vi "诊断标定4.vi"(8 "CAN端口":u16(ring), 9 "设备索引号":u16(ring), 10 "CAN卡类型":u32(ring)=4) -> ()   [LabVIEW 2013] (continued)
                  tunnel: w1914 -> [w1917 w1925]
                  tunnel: w1913 -> [w1916 w1924]
                  tunnel: w1912 -> [w1915 w1923]
                  tunnel: u8 137 ("命令") -> [_ w1922]
                  frame #0 {
                    n1213 = dll-call lib="PTH1Aabs EEV05EV05监控上位机-EV05EV05data\nusbcan.dll" fn="VCI_ClearBuffer"("DeviceType"=w1917, "DeviceInd"=w1916, "CANInd"=w1915) -> (error out=w1918:errorcluster)  [unwired: 4 in, 4 out]
                    n1214 = call <vilib>:"Clear Errors.vi"("error in (no error)"=w1918) -> ()  [unwired: 6 in, 1 out]
                  }
                  frame #1 {
                    w1921 = u32 2 ("命令序号")
                    n1215 = local read "从板板号"() -> (w1919:u8)
                    n1216 = local write "命令"(w1922) -> ()
                    n1217 = call "多帧发送机制(EV05).vi"("can卡类型"=w1925, "设备索引号"=w1924, "CAN端口"=w1923, "命令"=w1922, "板号"=w1919, "命令序号"=w1921, "输入数据"=dbl[] [0.0]) -> ()  [unwired: 1 in, 12 out]
                    n1218 = local write "命令序号"(w1921) -> ()
                  }
                }
              }
              frame #1 {
                n1219 = while {
                  tunnel: [w1927] -> w1926
                  i -> [w1932]
                  stop <- w1929 stop-if-true
                  n1220 = global read "EV05全局变量1.vi" "写入超时"() -> (w1927:bool)
                  n1221 = Greater Or Equal?(x=w1932, y=25) -> (x >= y?=w1930:bool)
                  n1222 = Or(x=w1927, y=w1930) -> (x .or. y?=w1929:bool)
                  n1223 = Wait Until Next ms Multiple(millisecond multiple=u32 100 ("毫秒倍数")) -> ()  [unwired: 1 out]
                }
              }
              frame #2 {
                n1224 = case shown="假" w1933 {
                  frame False {
                    n1225 = control-ref of="结果"() -> (w1936:refnum<vi>)
                    n1226 = Concatenate Strings("平台软件版本" ("字符串"), "     读取失败" ("字符串")) -> (w1938:string)
                    n1227 = Build Array(w1938) -> (w1935:string[])
                    n1228 = call "表格编辑(版本读取).vi"("新元素/子数组"=w1935, "活动单元格:单元格背景色"=u32 16740749, "MCListbox引用句柄"=w1936) -> ()  [unwired: 9 out]
                  }
                  frame True {
                  }
                }
                n1229 = call <vilib>:"Unset Busy.vi"() -> ()  [unwired: 2 in, 10 out]
              }
            }
          }
          frame "模块软件版本读取" {
            n1230 = local read "模块软件版本"() -> (w1941:T16)
            n1231 = local read "从板板号"() -> (w1940:u8)
            n1232 = case shown="\"全部读取\"" w1941 {
              selector: w1941 -> [w1942 w1986]
              tunnel: w1940 -> [_ w1985]
              frame "BCUMCAL", Default {
                n1233 = stacked-sequence {
                  seq-local: [_ _ w1968 _] -> [_ _ _ w1975]
                  tunnel: w1942 -> [_ w1948 _ w1976]
                  frame #0 {
                    w1947 = FALSE ("写?")
                    n1234 = call <vilib>:"Set Busy.vi"("disable click? (T)"=FALSE) -> ()  [unwired: 3 in, 8 out]
                    n1235 = local write "写?"(w1947) -> ()
                    n1236 = global write "EV05全局变量1.vi" "流控帧 2"(TRUE ("流控帧 2")) -> ()
                    n1237 = global write "EV05全局变量1.vi" "写入超时"(w1947) -> ()
                    n1238 = local write "控制1"(TRUE ("控制1")) -> ()
                    n1239 = local write "消除"(TRUE ("消除")) -> ()
                  }
                  frame #1 {
                    n1240 = Quotient & Remainder(x=w1948, y=256) -> (x-y*floor(x/y)=w1949:i32, floor(x/y)=w1950:i32)
                    n1241 = Build Array(w1950, w1949, u8 0 ("板号")) -> (w1953:i32[])
                    n1242 = local read "设备索引号"() -> (w1955:u16)
                    n1243 = local read "CAN卡类型"() -> (w1956:u32)
                    n1244 = local read "CAN端口"() -> (w1954:u16)
                    n1245 = stacked-sequence {
                      tunnel: w1956 -> [w1959 w1967]
                      tunnel: w1955 -> [w1958 w1966]
                      tunnel: w1954 -> [w1957 w1965]
                      tunnel: w1953 -> [_ w1964]
                      frame #0 {
                        n1246 = dll-call lib="PTH1Aabs EEV05EV05监控上位机-EV05EV05data\nusbcan.dll" fn="VCI_ClearBuffer"("DeviceType"=w1959, "DeviceInd"=w1958, "CANInd"=w1957) -> (error out=w1960:errorcluster)  [unwired: 4 in, 4 out]
                        n1247 = call <vilib>:"Clear Errors.vi"("error in (no error)"=w1960) -> ()  [unwired: 6 in, 1 out]
                      }
                      frame #1 {
                        w1963 = u8 137 ("命令")
                        w1961 = u32 3 ("命令序号")
                        n1248 = local read "从板板号"() -> (w1962:u8)
                        n1249 = local write "命令"(w1963) -> ()
                        n1250 = call "多帧发送机制(EV05).vi"("can卡类型"=w1967, "设备索引号"=w1966, "CAN端口"=w1965, "命令"=w1963, "板号"=w1962, "命令序号"=w1961, "输入数据"=w1964) -> ()  [unwired: 1 in, 12 out]
                        n1251 = local write "命令序号"(w1961) -> ()
                      }
                    }
                  }
                  frame #2 {
                    n1252 = while {
                      tunnel: [w1969] -> w1968
                      i -> [w1974]
                      stop <- w1970 stop-if-true
                      n1253 = global read "EV05全局变量1.vi" "写入超时"() -> (w1969:bool)
                      n1254 = Greater Or Equal?(x=w1974, y=25) -> (x >= y?=w1971:bool)
                      n1255 = Or(x=w1969, y=w1971) -> (x .or. y?=w1970:bool)
                      n1256 = Wait Until Next ms Multiple(millisecond multiple=u32 100 ("毫秒倍数")) -> ()  [unwired: 1 out]
                    }
                  }
                  frame #3 {
                    n1257 = call <vilib>:"Unset Busy.vi"() -> ()  [unwired: 2 in, 10 out]
                    n1258 = case shown="假" w1975 {
                      tunnel: w1976 -> [w1978 _]
                      frame False {
                        n1259 = Number To Decimal String(number=w1978) -> (decimal integer string=w1979:string)  [unwired: 1 out]
                        n1260 = control-ref of="结果"() -> (w1980:refnum<vi>)
                        n1261 = Concatenate Strings("模块" ("字符串"), w1979, "     读取失败" ("字符串")) -> (w1983:string)
                        n1262 = Build Array(w1983) -> (w1982:string[])
                        n1263 = call "表格编辑(版本读取).vi"("新元素/子数组"=w1982, "活动单元格:单元格背景色"=u32 16740749, "MCListbox引用句柄"=w1980) -> ()  [unwired: 9 out]
                      }
                      frame True {
                      }
                    }
                  }
                }
              }
              frame "全部读取" {
                n1264 = stacked-sequence {
                  seq-local: [w1987 _] -> [_ w2025]
                  tunnel: w1986 -> [_ w2027]
                  tunnel: w1985 -> [w1988 w2026]
                  frame #0 {
                    n1265 = stacked-sequence {
                      tunnel: w1988 -> [_ w1997 _]
                      tunnel: [_ _ w2017] -> w1987
                      frame #0 {
                        w1993 = FALSE ("写?")
                        n1266 = control-ref of="模块软件版本"() -> (w1991:refnum<vi>)
                        n1267 = call <vilib>:"Set Busy.vi"("disable click? (T)"=FALSE) -> ()  [unwired: 3 in, 8 out]
                        n1268 = local write "写?"(w1993) -> ()
                        n1269 = property class="MCListbox (严格)"(reference=w1991, "ItemNames"=string[][] []) -> ()  [unwired: 1 in, 2 out]
                        n1270 = global write "EV05全局变量1.vi" "写入超时"(w1993) -> ()
                        n1271 = global write "EV05全局变量1.vi" "流控帧 2"(TRUE ("流控帧 2")) -> ()
                        n1272 = local write "消除"(TRUE ("消除")) -> ()
                        n1273 = local write "控制1"(TRUE ("控制1")) -> ()
                        n1274 = local write "MODEL号"(u8[] [] ("MODEL号")) -> ()
                      }
                      frame #1 {
                        n1275 = local read "设备索引号"() -> (w1999:u16)
                        n1276 = local read "CAN卡类型"() -> (w2000:u32)
                        n1277 = local read "CAN端口"() -> (w1998:u16)
                        n1278 = stacked-sequence {
                          tunnel: w2000 -> [w2003 w2016]
                          tunnel: w1999 -> [w2002 w2015]
                          tunnel: w1998 -> [w2001 w2014]
                          tunnel: w1997 -> [_ w2006]
                          frame #0 {
                            n1279 = dll-call lib="PTH1Aabs EEV05EV05监控上位机-EV05EV05data\nusbcan.dll" fn="VCI_ClearBuffer"("DeviceType"=w2003, "DeviceInd"=w2002, "CANInd"=w2001) -> (error out=w2004:errorcluster)  [unwired: 4 in, 4 out]
                            n1280 = call <vilib>:"Clear Errors.vi"("error in (no error)"=w2004) -> ()  [unwired: 6 in, 1 out]
                          }
                          frame #1 {
                            w2012 = u8 137 ("命令")
                            w2010 = u32 3 ("命令序号")
                            n1281 = Quotient & Remainder(x=u8 0 ("板号"), y=256) -> (x-y*floor(x/y)=w2007:i32, floor(x/y)=w2008:i32)
                            n1282 = local write "命令"(w2012) -> ()
                            n1283 = Build Array(w2008, w2007, u8 0 ("板号")) -> (w2013:i32[])
                            n1284 = call "多帧发送机制(EV05).vi"("can卡类型"=w2016, "设备索引号"=w2015, "CAN端口"=w2014, "命令"=w2012, "板号"=w2006, "命令序号"=w2010, "输入数据"=w2013) -> ()  [unwired: 1 in, 12 out]
                            n1285 = local write "命令序号"(w2010) -> ()
                          }
                        }
                      }
                      frame #2 {
                        n1286 = while {
                          tunnel: [w2019] -> w2017
                          i -> [w2023]
                          stop <- w2020 stop-if-true
                          n1287 = local read "整车CAN测试"() -> (w2018:bool)
                          n1288 = global read "EV05全局变量1.vi" "写入超时"() -> (w2019:bool)
                          n1289 = Greater Or Equal?(x=w2023, y=35) -> (x >= y?=w2021:bool)
                          n1290 = Compound Arithmetic op=OR(w2018, w2019, w2021) -> (w2020:bool)
                          n1291 = Wait Until Next ms Multiple(millisecond multiple=u32 100 ("毫秒倍数")) -> ()  [unwired: 1 out]
                        }
                      }
                    }
                  }
                  frame #1 {
                    n1292 = case shown="真" w2025 {
                      tunnel: w2027 -> [_ w2037]
                      tunnel: w2026 -> [_ w2036]
                      frame False {
                        n1293 = control-ref of="结果"() -> (w2029:refnum<vi>)
                        n1294 = Concatenate Strings("模块编号" ("字符串"), "读取失败" ("字符串")) -> (w2032:string)
                        n1295 = Build Array(w2032) -> (w2031:string[])
                        n1296 = call "表格编辑(版本读取).vi"("新元素/子数组"=w2031, "活动单元格:单元格背景色"=u32 16740749, "MCListbox引用句柄"=w2029) -> ()  [unwired: 9 out]
                        n1297 = call <vilib>:"Unset Busy.vi"() -> ()  [unwired: 11 in, 1 out]
                      }
                      frame True {
                        n1298 = local read "MODEL号"() -> (w2035:u8[])
                        n1299 = Array Size(array=w2035) -> (size(s)=w2034:i32)
                        n1300 = for {
                          tunnel: w2037 -> [_]
                          tunnel: w2036 -> [w2040]
                          tunnel: w2035 -> [w2039] mode=indexing
                          tunnel: w2034 -> [w2038]
                          i -> [w2042]
                          n1301 = Increment(x=w2042) -> (x+1=w2041:i32)
                          n1302 = stacked-sequence {
                            seq-local: [_ _ _ w2069 _ _] -> [_ _ _ _ w2078 _]
                            seq-local: [_ w2048 _ _ _ _] -> [_ _ _ _ w2077 _]
                            tunnel: w2041 -> [_ _ _ _ _ w2089]
                            tunnel: w2039 -> [_ w2048 _ _ _ _]
                            tunnel: w2040 -> [_ w2049 _ _ _ _]
                            tunnel: w2038 -> [_ _ _ _ _ w2087]
                            frame #0 {
                              w2044 = FALSE ("写?")
                              n1303 = call <vilib>:"Set Busy.vi"("disable click? (T)"=FALSE) -> ()  [unwired: 3 in, 8 out]
                              n1304 = local write "写?"(w2044) -> ()
                              n1305 = global write "EV05全局变量1.vi" "写入超时"(w2044) -> ()
                              n1306 = global write "EV05全局变量1.vi" "流控帧 2"(TRUE ("流控帧 2")) -> ()
                              n1307 = local write "控制1"(TRUE ("控制1")) -> ()
                              n1308 = local write "消除"(TRUE ("消除")) -> ()
                            }
                            frame #1 {
                              n1309 = local read "设备索引号"() -> (w2051:u16)
                              n1310 = local read "CAN卡类型"() -> (w2052:u32)
                              n1311 = local read "CAN端口"() -> (w2050:u16)
                              n1312 = stacked-sequence {
                                tunnel: w2052 -> [w2055 w2068]
                                tunnel: w2051 -> [w2054 w2067]
                                tunnel: w2050 -> [w2053 w2066]
                                tunnel: w2049 -> [_ w2058]
                                tunnel: w2048 -> [_ w2057]
                                frame #0 {
                                n1313 = dll-call lib="PTH1Aabs EEV05EV05监控上位机-EV05EV05data\nusbcan.dll" fn="VCI_ClearBuffer"("DeviceType"=w2055, "DeviceInd"=w2054, "CANInd"=w2053) -> (error out=w2056:errorcluster)  [unwired: 4 in, 4 out]
                                n1314 = call <vilib>:"Clear Errors.vi"("error in (no error)"=w2056) -> ()  [unwired: 6 in, 1 out]
                                }
                                frame #1 {
                                w2064 = u8 137 ("命令")
                                w2062 = u32 3 ("命令序号")
                                n1315 = Quotient & Remainder(x=w2057, y=256) -> (x-y*floor(x/y)=w2059:i32, floor(x/y)=w2060:i32)
                                n1316 = local write "命令"(w2064) -> ()
                                n1317 = Build Array(w2060, w2059, u8 0 ("板号")) -> (w2065:i32[])
                                n1318 = call "多帧发送机制(EV05).vi"("can卡类型"=w2068, "设备索引号"=w2067, "CAN端口"=w2066, "命令"=w2064, "板号"=w2058, "命令序号"=w2062, "输入数据"=w2065) -> ()  [unwired: 1 in, 12 out]
                                n1319 = local write "命令序号"(w2062) -> ()
                                }
                              }
                            }
                            frame #2 {
                            }
                            frame #3 {
                              n1320 = while {
                                tunnel: [w2071] -> w2069
                                i -> [w2075]
                                stop <- w2072 stop-if-true
                                n1321 = local read "整车CAN测试"() -> (w2070:bool)
                                n1322 = global read "EV05全局变量1.vi" "写入超时"() -> (w2071:bool)
                                n1323 = Greater Or Equal?(x=w2075, y=25) -> (x >= y?=w2073:bool)
                                n1324 = Compound Arithmetic op=OR(w2070, w2071, w2073) -> (w2072:bool)
                                n1325 = Wait Until Next ms Multiple(millisecond multiple=u32 100 ("毫秒倍数")) -> ()  [unwired: 1 out]
                              }
                            }
                            frame #4 {
                              n1326 = call <vilib>:"Unset Busy.vi"() -> ()  [unwired: 11 in, 1 out]
                              n1327 = case shown="假" w2078 {
                                tunnel: w2077 -> [w2080 _]
                                frame False {
                                n1328 = control-ref of="结果"() -> (w2082:refnum<vi>)
                                n1329 = Number To Decimal String(number=w2080) -> (decimal integer string=w2081:string)  [unwired: 1 out]
                                n1330 = Concatenate Strings("模块" ("字符串"), w2081, "     读取失败" ("字符串")) -> (w2085:string)
                                n1331 = Build Array(w2085) -> (w2084:string[])
                                n1332 = call "表格编辑(版本读取).vi"("新元素/子数组"=w2084, "活动单元格:单元格背景色"=u32 16740749, "MCListbox引用句柄"=w2082) -> ()  [unwired: 9 out]
                                }
                                frame True {
                                }
                              }
                            }
                            frame #5 {
                              n1333 = Equal?(x=w2087, y=w2089) -> (x = y?=w2088:bool)
                              n1334 = case shown="真" w2088 {
                                frame False {
                                }
                                frame True {
                                n1335 = control-ref of="模块软件版本"() -> (w2100:refnum<vi>)
                                n1336 = local read "模块版本名称"() -> (w2099:string[][])
                                n1337 = local read "模块版本值"() -> (w2095:string[][])
                                n1338 = control-ref of="结果"() -> (w2107:refnum<vi>)
                                n1339 = property class="MCListbox (严格)"(reference=w2100) -> ("ItemNames"=w2103:string[][])  [unwired: 1 in, 2 out]
                                n1340 = local read "从板板号"() -> (w2090:u8)
                                n1341 = Concatenate Strings("模块版本读取完成" ("字符串")) -> (w2110:string)
                                n1342 = Build Array(w2110) -> (w2109:string[])
                                n1343 = call "表格编辑(版本读取).vi"("新元素/子数组"=w2109, "活动单元格:单元格背景色"=u32 21937, "MCListbox引用句柄"=w2107) -> ()  [unwired: 9 out]
                                n1344 = Transpose 2D Array(2D array=w2103) -> (transposed array=w2104:string[][])
                                n1345 = local read "模块个数"() -> (w2093:u8[])
                                n1346 = local write "整车CAN测试"(FALSE ("强制停止 2")) -> ()
                                n1347 = Index Array(array=w2104, index (row) #1=0 ("索引 (行)"), index (row) #2=1 ("索引 (行)")) -> (element #1=w2094:string[], element #2=w2096:string[])  [unwired: 2 in]
                                n1348 = Replace Array Subset(array=w2099, new element=w2094, index (row)=w2090) -> (w2098:string[][])  [unwired: 1 in]
                                n1349 = Replace Array Subset(array=w2095, new element=w2096, index (row)=w2090) -> (w2097:string[][])  [unwired: 1 in]
                                n1350 = local write "模块版本名称"(w2098) -> ()
                                n1351 = local write "模块版本值"(w2097) -> ()
                                n1352 = Array Size(array=w2094) -> (size(s)=w2091:i32)
                                n1353 = Replace Array Subset(array=w2093, new element=w2091, index=w2090) -> (w2092:u8[])
                                n1354 = local write "模块个数"(w2092) -> ()
                                }
                              }
                            }
                          }
                        }
                      }
                    }
                  }
                }
              }
            }
          }
          frame "硬件版本读取" {
            n1355 = stacked-sequence {
              seq-local: [_ _ w2118 _] -> [_ _ _ w2125]
              frame #0 {
                w2114 = u8 137 ("命令")
                w2113 = u32 4 ("命令序号")
                n1356 = local read "设备索引号"() -> (w2116:u16)
                n1357 = local read "CAN卡类型"() -> (w2117:u32)
                n1358 = local read "CAN端口"() -> (w2115:u16)
                n1359 = local read "从板板号"() -> (w2111:u8)
                n1360 = local write "命令"(w2114) -> ()
                n1361 = call "多帧发送机制(EV05).vi"("can卡类型"=w2117, "设备索引号"=w2116, "CAN端口"=w2115, "命令"=w2114, "板号"=w2111, "命令序号"=w2113, "输入数据"=dbl[] [0.0]) -> ()  [unwired: 1 in, 12 out]
                n1362 = local write "命令序号"(w2113) -> ()
              }
              frame #1 {
              }
              frame #2 {
                n1363 = while {
                  tunnel: [w2119] -> w2118
                  i -> [w2124]
                  stop <- w2120 stop-if-true
                  n1364 = global read "EV05全局变量1.vi" "写入超时"() -> (w2119:bool)
                  n1365 = Greater Or Equal?(x=w2124, y=25) -> (x >= y?=w2121:bool)
                  n1366 = Or(x=w2119, y=w2121) -> (x .or. y?=w2120:bool)
                  n1367 = Wait Until Next ms Multiple(millisecond multiple=u32 100 ("毫秒倍数")) -> ()  [unwired: 1 out]
                }
              }
              frame #3 {
                n1368 = case shown="假" w2125 {
                  frame False {
                    n1369 = control-ref of="结果"() -> (w2127:refnum<vi>)
                    n1370 = Concatenate Strings("硬件版本" ("字符串"), "     读取失败" ("字符串")) -> (w2130:string)
                    n1371 = Build Array(w2130) -> (w2129:string[])
                    n1372 = call "表格编辑(版本读取).vi"("新元素/子数组"=w2129, "活动单元格:单元格背景色"=u32 16740749, "MCListbox引用句柄"=w2127) -> ()  [unwired: 9 out]
                  }
                  frame True {
                  }
                }
                n1373 = call <vilib>:"Unset Busy.vi"() -> ()  [unwired: 2 in, 10 out]
              }
            }
          }
          frame "写配置文件" {
            n1374 = disable-structure shown="启用" {
              frame Enabled {
                n1375 = local read "主从选择"() -> (w2138:enum32{"主板", "从板"})
                n1376 = case shown="\"从板\"" w2138 {
                  tunnel: [w2156 w2339] -> w2141
                  tunnel: ["M0" w2345] -> w2139
                  frame "主板", Default {
                    n1377 = stacked-sequence {
                      seq-local: [w2161 _ _ _ _ _ _] -> [_ w2190 _ _ _ _ _]
                      seq-local: [string[] ["电池额定容量", "电池实际容量", "SOC", "SOH", "车牌号", "配置文件版本", "产品编号", "系统时钟"] _ _ _ _ _ _] -> [_ w2192 _ _ _ _ _]
                      seq-local: [_ _ _ _ string[] ["风机开启温度", "风机关闭温度", "加热开启温度", "加热关闭温度", "风机开启温差", "风机关闭温差", "加热关闭温差"] _ _] -> [_ _ _ _ _ w2291 _]
                      seq-local: [_ _ _ _ w2272 _ _] -> [_ _ _ _ _ w2289 _]
                      tunnel: [w2162 _ _ _ _ _ _] -> w2158
                      tunnel: [_ w2193 _ _ _ _ _] -> w2155
                      tunnel: [_ _ w2217 _ _ _ _] -> w2154
                      tunnel: [_ _ _ w2244 _ _ _] -> w2153
                      tunnel: [_ _ _ _ _ w2292 _] -> w2152
                      tunnel: [_ _ _ _ _ _ w2309] -> w2151
                      frame #0 {
                        n1378 = local read "从板个数"() -> (w2181:dbl)
                        n1379 = control-ref of="项目信息"() -> (w2182:refnum<vi>)
                        n1380 = control-ref of="项目信息2"() -> (w2175:refnum<vi>)
                        n1381 = property class="Clust (严格)"(reference=w2175) -> ("Value"=w2174:T8)  [unwired: 1 in, 2 out]
                        n1382 = property class="Tbl (严格)"(reference=w2182) -> ("Value"=w2178:string[][])  [unwired: 1 in, 2 out]
                        n1383 = Number To Decimal String(number=w2181) -> (decimal integer string=w2180:string)  [unwired: 1 out]
                        n1384 = Unbundle(w2174) -> ("电池额定容量(A)"=w2173:dbl, "电池实际容量(A)"=w2172:dbl, "车架(牌)号"=w2170:string, "配置文件版本"=w2169:string, "SOH(%)"=w2164:dbl, "SOC(%)"=w2163:dbl, "产品编号"=w2168:string, "系统时钟"=w2167:string)  [unwired: 1 out]
                        n1385 = Build Array("从板个数" ("元素"), w2180) -> (w2176:string[])
                        n1386 = Build Array(w2173, w2172, w2163, w2164) -> (w2171:dbl[])
                        n1387 = Build Array(w2170, w2169, w2168, w2167) -> (w2165:string[])
                        n1388 = Insert Into Array(array=w2178, index (row)=0 ("索引 (行)"), new element=w2176) -> (w2162:string[][])  [unwired: 1 in]
                        n1389 = for {
                          tunnel: w2171 -> [w2184] mode=indexing
                          tunnel: [w2183] -> w2166 mode=indexing
                          n1390 = Format Into String(format string="%#f" ("格式字符串"), w2184) -> (resulting string=w2183:string)  [unwired: 2 in, 1 out]
                        }
                        n1391 = Insert Into Array(array=w2166, new element=w2165) -> (w2161:string[])  [unwired: 1 in]
                      }
                      frame #1 {
                        n1392 = control-ref of="一级故障"() -> (w2213:refnum<vi>)
                        n1393 = property class="Clust (严格)"(reference=w2213) -> ("Value"=w2212:T9)  [unwired: 1 in, 2 out]
                        n1394 = Unbundle(w2212) -> ("总电压过高"=w2211:dbl, "整组电压不均衡"=w2206:dbl, "SOC过高"=w2199:dbl, "单体电压过高"=w2202:dbl, "总电压过低"=w2210:dbl, "温度过高"=w2209:dbl, "温度过低"=w2208:dbl, "单组电压不均衡"=w2207:dbl, "整组温度不均衡"=w2204:dbl, "单组温度不均衡"=w2205:dbl, "单体电压过低"=w2203:dbl, "充电电流过高"=w2201:dbl, "放电电流过高"=w2200:dbl, "SOC过低"=w2198:dbl, "内阻过大"=w2197:dbl, "极柱温度过高"=w2196:dbl, "SOH过低"=w2195:dbl)
                        n1395 = Build Array(w2211, w2210, w2209, w2208, w2207, w2206, w2205, w2204, w2202, w2203, w2201, w2200, w2199, w2198, w2197, w2196, w2195) -> (w2194:dbl[])
                        n1396 = for {
                          tunnel: w2194 -> [w2215] mode=indexing
                          tunnel: [w2214] -> w2189 mode=indexing
                          n1397 = Format Into String(format string="%#f" ("格式字符串"), w2215) -> (resulting string=w2214:string)  [unwired: 2 in, 1 out]
                        }
                        n1398 = Insert Into Array(array=w2190, new element=w2189) -> (w2188:string[])  [unwired: 1 in]
                        n1399 = Insert Into Array(array=w2192, new element=string[] ["总电压过高一级", "总电压过低一级", "温度过高一级", "温度过低一级", "单组电压不均衡一级", "整组电压不均衡一级", "单组温度不均衡一级", "整组温度不均衡一级", "单体电压过高一级", "单体电压过低一级", "充电电流过高一级", "放电电流过高一级", "SOC过高一级", "SOC过低一级", "内阻过大一级", "极柱温度过高一级", "SOH过低一级"]) -> (w2187:string[])  [unwired: 1 in]
                        n1400 = Build Array(w2187, w2188) -> (w2186:string[][])
                        n1401 = Transpose 2D Array(2D array=w2186) -> (transposed array=w2193:string[][])
                      }
                      frame #2 {
                        n1402 = control-ref of="一级故障 2"() -> (w2218:refnum<vi>)
                        n1403 = property class="Clust (严格)"(reference=w2218) -> ("Value"=w2240:T9)  [unwired: 1 in, 2 out]
                        n1404 = Unbundle(w2240) -> ("总电压过高"=w2239:dbl, "整组电压不均衡"=w2234:dbl, "SOC过高"=w2227:dbl, "单体电压过高"=w2230:dbl, "总电压过低"=w2238:dbl, "温度过高"=w2237:dbl, "温度过低"=w2236:dbl, "单组电压不均衡"=w2235:dbl, "整组温度不均衡"=w2232:dbl, "单组温度不均衡"=w2233:dbl, "单体电压过低"=w2231:dbl, "充电电流过高"=w2229:dbl, "放电电流过高"=w2228:dbl, "SOC过低"=w2226:dbl, "内阻过大"=w2225:dbl, "极柱温度过高"=w2224:dbl, "SOH过低"=w2223:dbl)
                        n1405 = Build Array(w2239, w2238, w2237, w2236, w2235, w2234, w2233, w2232, w2230, w2231, w2229, w2228, w2227, w2226, w2225, w2224, w2223) -> (w2222:dbl[])
                        n1406 = for {
                          tunnel: w2222 -> [w2242] mode=indexing
                          tunnel: [w2241] -> w2221 mode=indexing
                          n1407 = Format Into String(format string="%#f" ("格式字符串"), w2242) -> (resulting string=w2241:string)  [unwired: 2 in, 1 out]
                        }
                        n1408 = Build Array(string[] ["总电压过高二级", "总电压过低二级", "温度过高二级", "温度过低二级", "单组电压不均衡二级", "整组电压不均衡二级", "单组温度不均衡二级", "整组温度不均衡二级", "单体电压过高二级", "单体电压过低二级", "充电电流过高二级", "放电电流过高二级", "SOC过高二级", "SOC过低二级", "内阻过大二级", "极柱温度过高二级", "SOH过低二级"], w2221) -> (w2219:string[][])
                        n1409 = Transpose 2D Array(2D array=w2219) -> (transposed array=w2217:string[][])
                      }
                      frame #3 {
                        n1410 = control-ref of="一级故障 3"() -> (w2245:refnum<vi>)
                        n1411 = property class="Clust (严格)"(reference=w2245) -> ("Value"=w2267:T9)  [unwired: 1 in, 2 out]
                        n1412 = Unbundle(w2267) -> ("总电压过高"=w2266:dbl, "整组电压不均衡"=w2261:dbl, "SOC过高"=w2254:dbl, "单体电压过高"=w2257:dbl, "总电压过低"=w2265:dbl, "温度过高"=w2264:dbl, "温度过低"=w2263:dbl, "单组电压不均衡"=w2262:dbl, "整组温度不均衡"=w2259:dbl, "单组温度不均衡"=w2260:dbl, "单体电压过低"=w2258:dbl, "充电电流过高"=w2256:dbl, "放电电流过高"=w2255:dbl, "SOC过低"=w2253:dbl, "内阻过大"=w2252:dbl, "极柱温度过高"=w2251:dbl, "SOH过低"=w2250:dbl)
                        n1413 = Build Array(w2266, w2265, w2264, w2263, w2262, w2261, w2260, w2259, w2257, w2258, w2256, w2255, w2254, w2253, w2252, w2251, w2250) -> (w2249:dbl[])
                        n1414 = for {
                          tunnel: w2249 -> [w2269] mode=indexing
                          tunnel: [w2268] -> w2248 mode=indexing
                          n1415 = Format Into String(format string="%#f" ("格式字符串"), w2269) -> (resulting string=w2268:string)  [unwired: 2 in, 1 out]
                        }
                        n1416 = Build Array(string[] ["总电压过高三级", "总电压过低三级", "温度过高三级", "温度过低三级", "单组电压不均衡三级", "整组电压不均衡三级", "单组温度不均衡三级", "整组温度不均衡三级", "单体电压过高三级", "单体电压过低三级", "充电电流过高三级", "放电电流过高三级", "SOC过高三级", "SOC过低三级", "内阻过大三级", "极柱温度过高三级", "SOH过低三级"], w2248) -> (w2246:string[][])
                        n1417 = Transpose 2D Array(2D array=w2246) -> (transposed array=w2244:string[][])
                      }
                      frame #4 {
                        n1418 = control-ref of="加热控制参数"() -> (w2282:refnum<vi>)
                        n1419 = property class="Clust (严格)"(reference=w2282) -> ("Value"=w2281:T10)  [unwired: 1 in, 2 out]
                        n1420 = Unbundle(w2281) -> ("风机开启温度"=w2280:dbl, "风机关闭温度"=w2279:dbl, "加热开启温度"=w2278:dbl, "加热关闭温度"=w2277:dbl, "风机开启温差"=w2276:dbl, "风机关闭温差"=w2275:dbl, "加热关闭温差"=w2271:dbl)
                        n1421 = Build Array(w2280, w2279, w2278, w2277, w2276, w2275, w2271) -> (w2274:dbl[])
                        n1422 = for {
                          tunnel: w2274 -> [w2284] mode=indexing
                          tunnel: [w2283] -> w2272 mode=indexing
                          n1423 = Format Into String(format string="%#f" ("格式字符串"), w2284) -> (resulting string=w2283:string)  [unwired: 2 in, 1 out]
                        }
                      }
                      frame #5 {
                        n1424 = control-ref of="充电控制参数"() -> (w2302:refnum<vi>)
                        n1425 = property class="Clust (严格)"(reference=w2302) -> ("Value"=w2304:T11)  [unwired: 1 in, 2 out]
                        n1426 = Unbundle(w2304) -> ("最大允许单体电压"=w2301:dbl, "最大允许总电压"=w2300:dbl, "最小允许单体电压"=w2299:dbl, "最大允许充电电流"=w2298:dbl, "最小允许充电电流"=w2297:dbl, "最大允许充电温度"=w2296:dbl, "最小允许充电温度"=w2295:dbl, "电流步长"=w2294:dbl)
                        n1427 = Build Array(w2301, w2300, w2299, w2298, w2297, w2296, w2295, w2294) -> (w2303:dbl[])
                        n1428 = for {
                          tunnel: w2303 -> [w2306] mode=indexing
                          tunnel: [w2305] -> w2288 mode=indexing
                          n1429 = Format Into String(format string="%#f" ("格式字符串"), w2306) -> (resulting string=w2305:string)  [unwired: 2 in, 1 out]
                        }
                        n1430 = Insert Into Array(array=w2289, new element=w2288) -> (w2287:string[])  [unwired: 1 in]
                        n1431 = Insert Into Array(array=w2291, new element=string[] ["最大允许单体电压", "最大允许总电压", "最小允许单体电压", "最大允许充电电流", "最小允许充电电流", "最大允许充电温度", "最小允许充电温度", "电流步长"]) -> (w2286:string[])  [unwired: 1 in]
                        n1432 = Build Array(w2286, w2287) -> (w2293:string[][])
                        n1433 = Transpose 2D Array(2D array=w2293) -> (transposed array=w2292:string[][])
                      }
                      frame #6 {
                        n1434 = control-ref of="电池信息"() -> (w2330:refnum<vi>)
                        n1435 = property class="Clust (严格)"(reference=w2330) -> ("Value"=w2333:T12)  [unwired: 1 in, 2 out]
                        n1436 = Unbundle(w2333) -> ("电池串联"=w2329:dbl, "电池并联"=w2328:dbl, "累计放电总安时"=w2326:dbl, "电池包额定容量"=w2325:dbl, "电池包额定能量"=w2324:dbl, "电池包额定总电压"=w2323:dbl, "累计充电总安时"=w2327:dbl, "电池充满次数"=w2322:dbl, "电池放空次数"=w2321:dbl, "电池充电次数"=w2320:dbl, "电池生产日期"=w2318:string, "电池厂家"=w2317:string, "电池类型"=w2316:string, "电池包组号"=w2315:string, "电池包产权标识"=w2314:string, "电池应用车型"=w2313:string, "实际容量"=w2308:dbl)
                        n1437 = Build Array(w2318, w2317, w2316, w2315, w2314, w2313) -> (w2312:string[])
                        n1438 = Build Array(w2329, w2328, w2327, w2326, w2325, w2324, w2323, w2322, w2321, w2320, w2308) -> (w2319:dbl[])
                        n1439 = for {
                          tunnel: w2319 -> [w2335] mode=indexing
                          tunnel: [w2334] -> w2311 mode=indexing
                          n1440 = Format Into String(format string="%#f" ("格式字符串"), w2335) -> (resulting string=w2334:string)  [unwired: 2 in, 1 out]
                        }
                        n1441 = Insert Into Array(array=w2312, new element=w2311) -> (w2310:string[])  [unwired: 1 in]
                        n1442 = call <vilib>:"Unset Busy.vi"() -> ()  [unwired: 2 in, 10 out]
                        n1443 = Build Array(string[] ["电池生产日期", "电池厂商", "电池类型", "电池包组号", "电池包产权标识", "电池包应用车型", "电池串联", "电池并联", "累计充电总安时", "累计放电总安时", "电池包额定容量", "电池包额定能量", "电池包额定总电压", "电池充满次数", "电池放空次数", "电池充电次数", "实际容量"], w2310) -> (w2331:string[][])
                        n1444 = Transpose 2D Array(2D array=w2331) -> (transposed array=w2309:string[][])
                      }
                    }
                    n1445 = Insert Into Array(array=w2158, index (col)=2 ("禁用的索引 (列)"), new element #1=w2155, new element #2=w2154, new element #3=w2153, new element #4=w2152, new element #5=w2151) -> (w2156:string[][])  [unwired: 1 in]
                  }
                  frame "从板" {
                    n1446 = local read "从板板号"() -> (w2347:u8)
                    n1447 = Number To Decimal String(number=w2347) -> (decimal integer string=w2344:string)  [unwired: 1 out]
                    n1448 = Concatenate Strings("S", w2344) -> (w2345:string)
                    n1449 = Build Array("从板号" ("元素"), w2344) -> (w2342:string[])
                    n1450 = stacked-sequence {
                      seq-local: [string[] ["风机开启温度", "风机关闭温度", "加热开启温度", "加热关闭温度", "风机开启温差", "风机关闭温差", "加热关闭温差"] _ _ _ _] -> [_ _ _ w2407 _]
                      seq-local: [w2349 _ _ _ _] -> [_ _ _ w2403 _]
                      seq-local: [_ string[] ["电压过高一级", "电压过低一级", "温度过高一级", "温度过低一级", "电压不均衡一级", "温度不均衡一级", "SOC过低一级"] _ _ _] -> [_ _ _ w2406 _]
                      seq-local: [_ w2368 _ _ _] -> [_ _ _ w2402 _]
                      seq-local: [_ _ string[] ["电压过高二级", "电压过低二级", "温度过高二级", "温度过低二级", "电压不均衡二级", "温度不均衡二级", "SOC过低二级"] _ _] -> [_ _ _ w2405 _]
                      seq-local: [_ _ w2383 _ _] -> [_ _ _ w2401 _]
                      tunnel: w2342 -> [w2362 _ _ _ _]
                      tunnel: [w2351 _ _ _ _] -> w2340
                      tunnel: [_ _ _ w2408 _] -> w2338
                      tunnel: [_ _ _ _ w2441] -> w2337
                      frame #0 {
                        n1451 = control-ref of="项目信息 2"() -> (w2361:refnum<vi>)
                        n1452 = property class="Tbl (严格)"(reference=w2361) -> ("Value"=w2364:string[][])  [unwired: 1 in, 2 out]
                        n1453 = control-ref of="加热控制参数"() -> (w2353:refnum<vi>)
                        n1454 = property class="Clust (严格)"(reference=w2353) -> ("Value"=w2360:T10)  [unwired: 1 in, 2 out]
                        n1455 = Unbundle(w2360) -> ("风机开启温度"=w2359:dbl, "风机关闭温度"=w2358:dbl, "加热开启温度"=w2357:dbl, "加热关闭温度"=w2356:dbl, "风机开启温差"=w2355:dbl, "风机关闭温差"=w2354:dbl, "加热关闭温差"=w2348:dbl)
                        n1456 = Build Array(w2359, w2358, w2357, w2356, w2355, w2354, w2348) -> (w2352:dbl[])
                        n1457 = Insert Into Array(array=w2364, index (row)=0 ("索引 (行)"), new element=w2362) -> (w2351:string[][])  [unwired: 1 in]
                        n1458 = for {
                          tunnel: w2352 -> [w2366] mode=indexing
                          tunnel: [w2365] -> w2349 mode=indexing
                          n1459 = Format Into String(format string="%#f" ("格式字符串"), w2366) -> (resulting string=w2365:string)  [unwired: 2 in, 1 out]
                        }
                      }
                      frame #1 {
                        n1460 = control-ref of="一级故障(从板)"() -> (w2379:refnum<vi>)
                        n1461 = property class="Clust (严格)"(reference=w2379) -> ("Value"=w2378:T14)  [unwired: 1 in, 2 out]
                        n1462 = Unbundle(w2378) -> ("电压过高"=w2377:dbl, "电压过低"=w2376:dbl, "温度过高"=w2375:dbl, "温度过低"=w2374:dbl, "电压不均衡(V)"=w2373:dbl, "温度不均衡"=w2372:dbl, "SOC过低"=w2371:dbl)
                        n1463 = Build Array(w2377, w2376, w2375, w2374, w2373, w2372, w2371) -> (w2370:dbl[])
                        n1464 = for {
                          tunnel: w2370 -> [w2381] mode=indexing
                          tunnel: [w2380] -> w2368 mode=indexing
                          n1465 = Format Into String(format string="%#f" ("格式字符串"), w2381) -> (resulting string=w2380:string)  [unwired: 2 in, 1 out]
                        }
                      }
                      frame #2 {
                        n1466 = control-ref of="二级故障(从板)"() -> (w2385:refnum<vi>)
                        n1467 = property class="Clust (严格)"(reference=w2385) -> ("Value"=w2394:T14)  [unwired: 1 in, 2 out]
                        n1468 = Unbundle(w2394) -> ("电压过高"=w2393:dbl, "电压过低"=w2392:dbl, "温度过高"=w2391:dbl, "温度过低"=w2390:dbl, "电压不均衡(V)"=w2389:dbl, "温度不均衡"=w2388:dbl, "SOC过低"=w2387:dbl)
                        n1469 = Build Array(w2393, w2392, w2391, w2390, w2389, w2388, w2387) -> (w2386:dbl[])
                        n1470 = for {
                          tunnel: w2386 -> [w2396] mode=indexing
                          tunnel: [w2395] -> w2383 mode=indexing
                          n1471 = Format Into String(format string="%#f" ("格式字符串"), w2396) -> (resulting string=w2395:string)  [unwired: 2 in, 1 out]
                        }
                      }
                      frame #3 {
                        n1472 = control-ref of="三级故障(从板)"() -> (w2409:refnum<vi>)
                        n1473 = property class="Clust (严格)"(reference=w2409) -> ("Value"=w2419:T14)  [unwired: 1 in, 2 out]
                        n1474 = Unbundle(w2419) -> ("电压过高"=w2418:dbl, "电压过低"=w2417:dbl, "温度过高"=w2416:dbl, "温度过低"=w2415:dbl, "电压不均衡(V)"=w2414:dbl, "温度不均衡"=w2413:dbl, "SOC过低"=w2412:dbl)
                        n1475 = Build Array(w2418, w2417, w2416, w2415, w2414, w2413, w2412) -> (w2411:dbl[])
                        n1476 = for {
                          tunnel: w2411 -> [w2421] mode=indexing
                          tunnel: [w2420] -> w2400 mode=indexing
                          n1477 = Format Into String(format string="%#f" ("格式字符串"), w2421) -> (resulting string=w2420:string)  [unwired: 2 in, 1 out]
                        }
                        n1478 = Insert Into Array(array=w2407, new element #1=w2406, new element #2=w2405, new element #3=string[] ["电压过高三级", "电压过低三级", "温度过高三级", "温度过低三级", "电压不均衡三级", "温度不均衡三级", "SOC过低三级"]) -> (w2398:string[])  [unwired: 1 in]
                        n1479 = Insert Into Array(array=w2403, new element #1=w2402, new element #2=w2401, new element #3=w2400) -> (w2399:string[])  [unwired: 1 in]
                        n1480 = Build Array(w2398, w2399) -> (w2410:string[][])
                        n1481 = Transpose 2D Array(2D array=w2410) -> (transposed array=w2408:string[][])
                      }
                      frame #4 {
                        n1482 = control-ref of="快换(从板)"() -> (w2440:refnum<vi>)
                        n1483 = property class="Clust (严格)"(reference=w2440) -> ("Value"=w2453:T15)  [unwired: 1 in, 2 out]
                        n1484 = Unbundle(w2453) -> ("电池类型"=w2452:dbl, "电池厂家"=w2451:dbl, "电池地区"=w2450:dbl, "电池组序号"=w2449:dbl, "电池包串联数"=w2448:dbl, "电池包并联数"=w2447:dbl, "电池包安时数"=w2446:dbl, "电池包序号"=w2439:dbl, "充电次数"=w2438:dbl, "充满电时间"=w2437:dbl, "放空时间"=w2436:dbl, "车牌号"=w2430:string, "最大允许单体电压"=w2429:dbl, "最大允许总电压"=w2435:dbl, "最大允许温度"=w2434:dbl, "最小允许温度"=w2433:dbl, "最大允许充电电流"=w2432:dbl, "最小允许充电电流"=w2428:dbl, "最小允许单体电压"=w2427:dbl, "电流步长"=w2426:dbl, "SOC"=w2425:dbl, "充电总安时"=w2424:dbl, "放电总这时"=w2423:dbl)
                        n1485 = Build Array(w2452, w2451, w2450, w2449, w2448, w2447, w2446, w2439, w2438, w2437, w2436, w2429, w2435, w2434, w2433, w2432, w2428, w2427, w2426, w2425, w2424, w2423) -> (w2445:dbl[])
                        n1486 = for {
                          tunnel: w2445 -> [w2455] mode=indexing
                          tunnel: [w2454] -> w2443 mode=indexing
                          n1487 = Format Into String(format string="%#f" ("格式字符串"), w2455) -> (resulting string=w2454:string)  [unwired: 2 in, 1 out]
                        }
                        n1488 = Insert Into Array(array=w2443, new element=w2430) -> (w2431:string[])  [unwired: 1 in]
                        n1489 = call <vilib>:"Unset Busy.vi"() -> ()  [unwired: 2 in, 10 out]
                        n1490 = Build Array(string[] ["电池类型", "电池厂家", "电池地区", "电池组序号", "电池包串联数", "电池包并联数", "电池包安时数", "电池包序号", "充电次数", "充满电时间", "放空时间", "最大允许单体电压", "最大允许总电压", "最大允许温度", "最小允许温度", "最大允许充电电流", "最小允许充电电流", "最小允许单体电压", "电流步长", "SOC", "充电总安时", "放电总安时"], w2431) -> (w2444:string[][])
                        n1491 = Transpose 2D Array(2D array=w2444) -> (transposed array=w2441:string[][])
                      }
                    }
                    n1492 = Insert Into Array(array=w2340, index (col)=2 ("禁用的索引 (列)"), new element #1=w2338, new element #2=w2337) -> (w2339:string[][])  [unwired: 1 in]
                  }
                }
                n1493 = call "当前时间解析-8.6.vi"() -> ("名称格式时间"=w2140:string)  [unwired: 1 in, 18 out]
                n1494 = Concatenate Strings(w2140, w2139) -> (w2137:string)
                n1495 = call <vilib>:"Application Directory.vi"() -> ("Application Directory"=w2134:path)
                n1496 = call "文件对话框2"("start path"=w2134, "prompt"="选择保存的路径", "default name"=w2137) -> ("selected path"=w2135:path, "cancelled"=w2133:bool, "error out"=w2132:errorcluster)  [unwired: 9 in, 1 out]
                n1497 = call <vilib>:"Clear Errors.vi"("error in (no error)"=w2132) -> ()  [unwired: 6 in, 1 out]
                n1498 = case shown="假" w2133 {
                  tunnel: w2141 -> [w2146 _]
                  tunnel: w2135 -> [w2142 _]
                  frame False {
                    n1499 = call-poly <vilib>:"Write To Spreadsheet File.vi"("append to file? (new file:F)"=FALSE, "2D data"=w2146, "file path (dialog if empty)"=w2142) -> ("new file path (Not A Path if cancelled)"=w2144:path)  [unwired: 3 in, 2 out]
                    n1500 = Path To String(path=w2144) -> (string=w2143:string)
                    n1501 = stacked-sequence {
                      tunnel: w2143 -> [w2149]
                      frame #0 {
                        n1502 = Concatenate Strings("保存完成,路径为:" ("字符串"), w2149) -> (w2150:string)
                        n1503 = One Button Dialog(message=w2150, button name ("OK")="是" ("按钮名称（“确定”）")) -> ()  [unwired: 1 out]
                      }
                    }
                  }
                  frame True {
                  }
                }
              }
              frame Disabled {
                n1504 = stacked-sequence {
                  seq-local: [w2470] -> [_]
                  frame #0 {
                    n1505 = local read "项目信息"() -> (w2472:string[][])
                    n1506 = local read "一级故障 4"() -> (w2469:T8)
                    n1507 = Array Subset(array=w2472, index (row)=0 ("索引"), index (col)=0 ("索引"), length (col)=2 ("索引")) -> (w2475:string[][])  [unwired: 1 in]
                    n1508 = local read "一级故障"() -> ()  [unwired: 1 out]
                    n1509 = local read "从板个数"() -> (w2470:dbl)
                    n1510 = Unbundle(w2469) -> ("电池额定容量(A)"=w2468:dbl, "电池实际容量(A)"=w2467:dbl, "车架(牌)号"=w2461:string, "配置文件版本"=w2460:string, "SOH(%)"=w2465:dbl, "SOC(%)"=w2466:dbl, "产品编号"=w2462:string)  [unwired: 2 out]
                    n1511 = Index Array(array=w2475, index (col) #1=1 ("禁用的索引 (列)"), index (col) #2=0 ("索引 (列)")) -> (element #1=w2459:string[], element #2=w2458:string[])  [unwired: 2 in]
                    n1512 = Build Array(w2468, w2467, w2466, w2465) -> (w2464:dbl[])
                    n1513 = Number To Decimal String(number=w2470) -> ()  [unwired: 1 in, 1 out]
                    n1514 = for {
                      tunnel: w2464 -> [w2480] mode=indexing
                      tunnel: [w2479] -> w2463 mode=indexing
                      n1515 = Format Into String(format string="%#f" ("格式字符串"), w2480) -> (resulting string=w2479:string)  [unwired: 2 in, 1 out]
                    }
                    n1516 = Insert Into Array(array=w2463, new element #1=w2462, new element #2=w2461, new element #3=w2460, new element #4=w2459) -> ()  [unwired: 1 in, 1 out]
                    n1517 = Insert Into Array(array=string[] ["电池额定容量", "电池实际容量", "SOC", "SOH", "产品编号", "车架(牌)号", "配置文件版本"], new element=w2458) -> ()  [unwired: 1 in, 1 out]
                  }
                }
              }
            }
          }
          frame "读配置文件" {
            n1518 = local read "主从选择"() -> (w2492:enum32{"主板", "从板"})
            n1519 = case shown="\"主板\", 默认" w2492 {
              tunnel: ["M" ("pattern (all files)") "S" ("pattern (all files)")] -> _
              tunnel: ["主板" ("pattern (all files)") "从板" ("pattern (all files)")] -> w2491
              frame "主板", Default {
              }
              frame "从板" {
              }
            }
            n1520 = case shown="真" "布尔" {
              tunnel: [w2855 w2860] -> w2484
              tunnel: [FALSE ("cancelled") w2859] -> _
              tunnel: w2491 -> [_ w2858]
              frame False {
                n1521 = local read "路径"() -> (w2855:path)
              }
              frame True {
                n1522 = call <vilib>:"Application Directory.vi"() -> ("Application Directory"=w2857:path)
                n1523 = call "文件对话框"("start path"=w2857, "prompt"="选择要读取的配置文件", "button label"=w2858) -> ("selected path"=w2860:path, "cancelled"=w2859:bool, "error out"=w2856:errorcluster)  [unwired: 4 in, 6 out]
                n1524 = call <vilib>:"Clear Errors.vi"("error in (no error)"=w2856) -> ()  [unwired: 7 out]
              }
            }
            n1525 = control-ref of="结果"() -> (w2490:refnum<vi>)
            n1526 = Strip Path(path=w2484) -> (name=w2488:string)  [unwired: 1 out]
            n1527 = Match Pattern(string=w2488, regular expression=".ini" ("正则表达式")) -> (offset past match=w2486:i32)  [unwired: 1 in, 3 out]
            n1528 = Not Equal?(x=w2486, y=-1) -> (x != y?=w2481:bool)
            n1529 = case shown="真" w2481 {
              tunnel: w2484 -> [_ w2501]
              tunnel: [_ w2510] -> w2482
              frame False {
              }
              frame True {
                w2513 = "MD5码" ("key")
                w2514 = "总信息" ("section")
                n1530 = Strip Path(path=w2501) -> (stripped path=w2499:path, name=w2498:string)
                n1531 = Match Pattern(string=w2498, regular expression=".ini" ("正则表达式")) -> (before substring=w2495:string, match substring=w2496:string)  [unwired: 1 in, 2 out]
                n1532 = Concatenate Strings(w2495, "-rc" ("字符串"), w2496) -> (w2494:string)
                n1533 = Build Path(base path=w2499, name or relative path=w2494) -> (appended path=w2500:path)
                n1534 = Copy(10:w2500, 11:w2501) -> (3:w2505:path)  [unwired: 3 in, 2 out]
                n1535 = call <vilib>:"Open Config Data.vi"("create file if necessary (T)"=FALSE, "configuration file path"=w2505) -> ("refnum"=w2516:T22)  [unwired: 7 in, 2 out]
                n1536 = call-poly <vilib>:"Read Key.vi"("section"=w2514, "key"=w2513, "refnum"=w2516) -> ("value"=w2511:string, "refnum out"=w2515:T22)  [unwired: 5 in, 2 out]
                n1537 = call-poly <vilib>:"Write Key.vi"("section"=w2514, "value"=w2513, "key"=w2513, "refnum"=w2515) -> ("error out"=w2509:errorcluster, "found?"=w2508:bool, "refnum out"=w2507:T22)  [unwired: 5 in]
                n1538 = call <vilib>:"Close Config Data.vi"("error in (no error)"=w2509, "write file if changed (T)"=w2508, "refnum"=w2507) -> ("error out"=w2506:errorcluster, "file path"=w2503:path)  [unwired: 7 in]
                n1539 = call <vilib>:"MD5Checksum File.vi"("error in (no error)"=w2506, "Path"=w2503) -> ("error out"=w2504:errorcluster, "MD5 message-digest"=w2512:string)  [unwired: 8 in]
                n1540 = Equal?(x=w2512, y=w2511) -> (x = y?=w2510:bool)
                n1541 = Delete(path (use dialog)=w2503, error in=w2504) -> (error out=w2502:errorcluster)  [unwired: 3 in, 2 out]
                n1542 = call <vilib>:"Clear Errors.vi"("error in (no error)"=w2502) -> ()  [unwired: 6 in, 1 out]
              }
            }
            n1543 = And(x=w2481, y=w2482) -> (x .and. y?=w2483:bool)
            n1544 = case shown="真" w2483 {
              tunnel: w2484 -> [_ w2534]
              tunnel: w2490 -> [w2520 w2533]
              tunnel: w2482 -> [w2519 _]
              tunnel: w2481 -> [w2518 _]
              frame False {
                n1545 = stacked-sequence {
                  tunnel: w2518 -> [w2522 _]
                  tunnel: w2520 -> [w2521 w2528]
                  tunnel: w2519 -> [_ w2527]
                  frame #0 {
                    n1546 = case shown="假" w2522 {
                      tunnel: w2521 -> [w2524 _]
                      frame False {
                        n1547 = Build Array("文件格式错误") -> (w2525:string[])
                        n1548 = call "表格编辑.vi"("新元素/子数组"=w2525, "活动单元格:单元格背景色"=u32 16711680, "MCListbox引用句柄"=w2524) -> ()  [unwired: 9 out]
                      }
                      frame True {
                      }
                    }
                  }
                  frame #1 {
                    n1549 = case shown="假" w2527 {
                      tunnel: w2528 -> [w2530 _]
                      frame False {
                        n1550 = Build Array("文件MD5码验证错误") -> (w2531:string[])
                        n1551 = call "表格编辑.vi"("新元素/子数组"=w2531, "活动单元格:单元格背景色"=u32 16711680, "MCListbox引用句柄"=w2530) -> ()  [unwired: 9 out]
                      }
                      frame True {
                      }
                    }
                  }
                }
                n1552 = call <vilib>:"Unset Busy.vi"() -> ()  [unwired: 11 in, 1 out]
              }
              frame True {
                n1553 = stacked-sequence {
                  seq-local: [w2539 _ _ _] -> [_ w2757 w2824 _]
                  seq-local: [w2537 _ _ _] -> [_ w2735 _ _]
                  tunnel: w2534 -> [w2535 _ _ _]
                  tunnel: w2533 -> [w2552 _ _ w2849]
                  frame #0 {
                    w2536 = string[][] []
                    w2549 = "总信息" ("section")
                    n1554 = local write "路径"(w2535) -> ()
                    n1555 = call <vilib>:"Open Config Data.vi"("create file if necessary (T)"=FALSE, "configuration file path"=w2535) -> ("error out"=w2540:errorcluster, "refnum"=w2539:T22)  [unwired: 7 in, 1 out]
                    n1556 = call <vilib>:"Get Key Names.vi"("section"=w2549, "error in (no error)"=w2540, "refnum"=w2539) -> ("key names"=w2548:string[], "refnum out"=w2550:T22)  [unwired: 5 in, 2 out]
                    n1557 = for {
                      tunnel: w2550 -> [w2556]
                      tunnel: w2549 -> [w2555]
                      tunnel: w2548 -> [w2554] mode=indexing
                      tunnel: [w2553] -> w2545 mode=indexing
                      n1558 = call-poly <vilib>:"Read Key.vi"("section"=w2555, "key"=w2554, "refnum"=w2556) -> ("value"=w2553:string)  [unwired: 5 in, 3 out]
                    }
                    n1559 = Index Array(array=w2545) -> (element #1=w2538:string, element #2=w2543:string)  [unwired: 2 in]
                    n1560 = Decimal String To Number(string=w2538) -> (number=w2537:i32)  [unwired: 2 in, 1 out]
                    n1561 = Concatenate Strings("正在读取" ("字符串"), w2543, "的配置文件" ("字符串")) -> (w2541:string)
                    n1562 = Build Array(w2541) -> (w2546:string[])
                    n1563 = local write "项目信息"(w2536) -> ()
                    n1564 = local write "项目信息 2"(w2536) -> ()
                    n1565 = call "表格编辑.vi"("新元素/子数组"=w2546, "活动单元格:单元格背景色"=u32 6618880, "MCListbox引用句柄"=w2552) -> ()  [unwired: 9 out]
                  }
                  frame #1 {
                    w2717 = 20 ("长度")
                    w2758 = "主板" ("section")
                    n1566 = call <vilib>:"Get Key Names.vi"("section"=w2758, "refnum"=w2757) -> ("key names"=w2628:string[], "refnum out"=w2759:T22)  [unwired: 6 in, 2 out]
                    n1567 = for {
                      tunnel: w2759 -> [w2771]
                      tunnel: w2758 -> [w2770]
                      tunnel: w2628 -> [w2769] mode=indexing
                      tunnel: [w2768] -> w2595 mode=indexing
                      n1568 = call-poly <vilib>:"Read Key.vi"("section"=w2770, "key"=w2769, "refnum"=w2771) -> ("value"=w2768:string)  [unwired: 5 in, 3 out]
                    }
                    n1569 = Search 1D Array(1D array=w2628, element="总电压过高一级" ("元素"), start index (0)=0 ("开始索引(0)")) -> (index of element=w2639:i32)
                    n1570 = Search 1D Array(1D array=w2628, element="风机开启温度" ("元素"), start index (0)=w2639) -> (index of element=w2630:i32)
                    n1571 = Search 1D Array(1D array=w2628, element="电池串联" ("元素"), start index (0)=w2630) -> (index of element=w2627:i32)
                    n1572 = Decrement(x=w2639) -> (x-1=w2756:i32)
                    n1573 = Array Subset(array=w2628, index=1 ("索引"), length=w2756) -> (w2603:string[])
                    n1574 = Array Subset(array=w2595, index=1 ("索引"), length=w2756) -> (w2599:string[])
                    n1575 = Delete From Array(array=w2603, length=7 ("长度"), index=0 ("索引")) -> (array with subset deleted=w2602:string[])  [unwired: 1 out]
                    n1576 = Delete From Array(array=w2599, length=7 ("长度"), index=0 ("索引")) -> (deleted portion=w2594:string[], array with subset deleted=w2598:string[])
                    n1577 = Index Array(array=w2595, index=0 ("索引")) -> (element=w2732:string)
                    n1578 = Decimal String To Number(string=w2732) -> (number=w2571:i32)  [unwired: 2 in, 1 out]
                    n1579 = Search 1D Array(1D array=w2602, element="主板电池节数" ("元素")) -> (index of element=w2723:i32)  [unwired: 1 in]
                    n1580 = Search 1D Array(1D array=w2602, element="主板温度起始值" ("元素")) -> (index of element=w2720:i32)  [unwired: 1 in]
                    n1581 = Search 1D Array(1D array=w2602, element="第一个保险通道" ("元素")) -> (index of element=w2719:i32)  [unwired: 1 in]
                    n1582 = Search 1D Array(1D array=w2602, element="主板温度个数" ("元素")) -> (index of element=w2721:i32)  [unwired: 1 in]
                    n1583 = Search 1D Array(1D array=w2602, element="主板电压起始值" ("元素")) -> (index of element=w2722:i32)  [unwired: 1 in]
                    n1584 = Search 1D Array(1D array=w2602, element="第1通道电压个数" ("元素")) -> (index of element=w2718:i32)  [unwired: 1 in]
                    n1585 = for {
                      N: 4 -> [_]
                      tunnel: w2594 -> [w2767] mode=indexing
                      tunnel: [w2766] -> w2747 mode=indexing
                      n1586 = Fract/Exp String To Number(string=w2767) -> (number=w2766:dbl)  [unwired: 3 in, 1 out]
                    }
                    n1587 = Increment(x=w2571) -> (x+1=w2731:i32)
                    n1588 = Increment(x=w2571) -> (x+1=w2716:i32)
                    n1589 = Increment(x=w2571) -> (x+1=w2729:i32)
